vi "(SubVI) Get avg_fps.vi"(7 "TTB array (ms)\ntime axis (ms)":u32[](array[numeric])) -> (0 "med. fps (Hz)":dbl, 1 "avg. fps (Hz)":dbl, 2 "Time Axis (s)":dbl[](array[numeric]), 3 "acquire time array (ms)":u32[](array[numeric]))   [LabVIEW 2014]
uses:
  <vilib>/Analysis/baseanly.llb/Mean (DBL).vi
  <vilib>/Analysis/NI_AALBase.lvlib
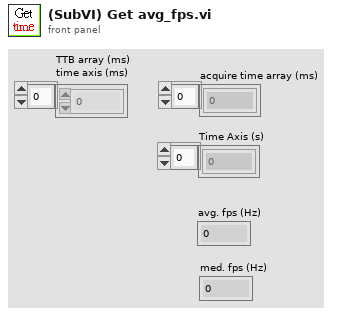
[diagram p1: front panel]
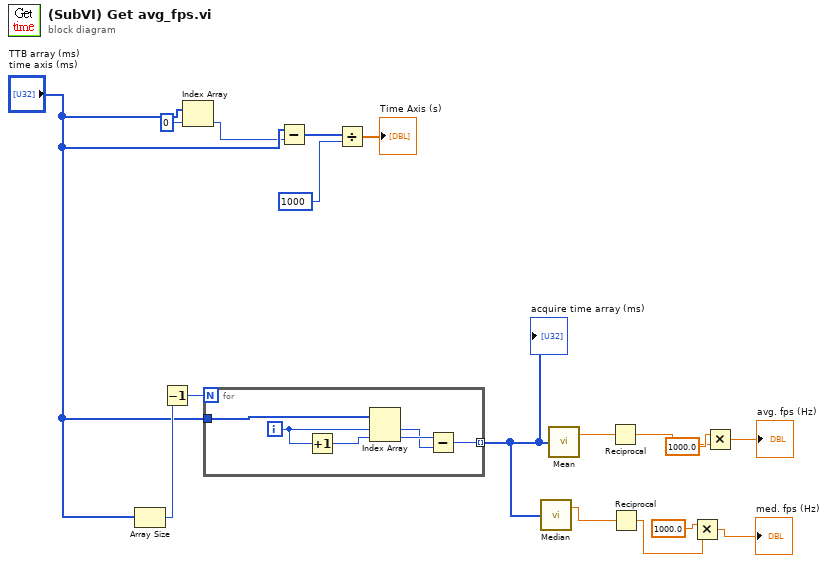
[diagram p0: block diagram]
diagram:
  n1 = Array Size(array="TTB array (ms)\ntime axis (ms)") -> (size(s)=w12:i32)
  n2 = Decrement(x=w12) -> (x-1=w13:i32)
  n3 = Index Array(array="TTB array (ms)\ntime axis (ms)", index=0) -> (element=w4:u32)
  n4 = for {
    N: w13 -> [_]
    tunnel: "TTB array (ms)\ntime axis (ms)" -> [w23]
    tunnel: [w18] -> w11 mode=indexing
    i -> [w22]
    n5 = Increment(x=w22) -> (x+1=w21:i32)
    n6 = Index Array(array=w23, index #1=w22, index #2=w21) -> (element #1=w19:u32, element #2=w20:u32)
    n7 = Subtract(x=w20, y=w19) -> (x-y=w18:u32)
  }
  "acquire time array (ms)" <- w11
  n8 = Subtract(x="TTB array (ms)\ntime axis (ms)", y=w4) -> (x-y=w3:u32[])
  n9 = Divide(x=w3, y=1000 ("index")) -> (x/y=→"Time Axis (s)":dbl[])
  n10 = call <vilib>:"Median.vi"("X"=w11) -> ("median"=w9:dbl)  [unwired: 1 out]
  n11 = call-poly <vilib>:"Mean.vi"("X"=w11) -> ("mean"=w14:dbl)  [unwired: 1 out]
  n12 = Reciprocal(x=w14) -> (1/x=w15:dbl)
  n13 = Reciprocal(x=w9) -> (1/x=w8:dbl)
  n14 = Multiply(x=1000.0 ("y"), y=w8) -> (x*y=→"med. fps (Hz)":dbl)
  n15 = Multiply(x=1000.0 ("y"), y=w15) -> (x*y=→"avg. fps (Hz)":dbl)
